vi "Solve2.vi"(8 "Error In":errorcluster, 11 "object in":refnum<class "2024_11.lvclass">) -> (0 "Error Out":errorcluster, 2 "Result":u64, 3 "object out":refnum<class "2024_11.lvclass">)   [LabVIEW 2023, in "2024_11.lvclass"]
uses:
  2024_11.lvclass
  2024_11.lvclass/2024_11.ctl
panel:
  out "x-y":u32
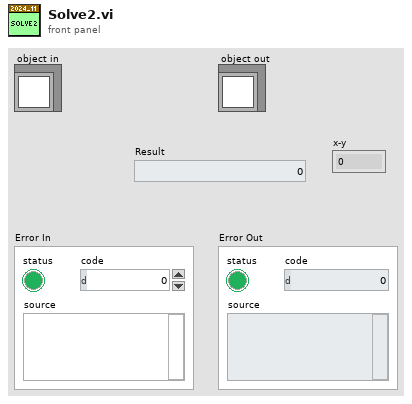
[diagram p1: front panel]
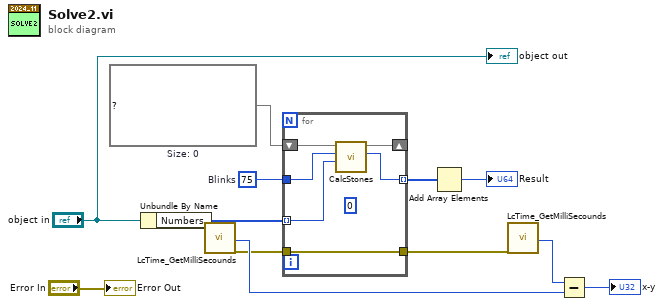
[diagram p0: block diagram]
diagram:
  w6 = 75  # Blinks
  w7 = map{cluster{"Number":u64, "Blinks":i32}, u64} {}  # Size: 0
  n1 = Unbundle By Name("object in") -> ("Numbers"=w10:u64[])
  n2 = call <userlib>:"LcTime_GetMilliSecounds.vi"() -> ("msValue"=w4:u32, "error out"=w2:errorcluster)  [unwired: 18 in]
  n3 = for {
    tunnel: w10 -> [w17] mode=indexing
    tunnel: [w15] -> w8 mode=indexing
    shift-right: [w16] -> _
    shift-left: w7 -> [w18]
    tunnel: w6 -> [w14]
    tunnel: w2 -> [w13]
    tunnel: [w13] -> w1
    (unwired) 0
    n4 = call "CalcStones.vi"("StoneNumber"=w17, "BlinkNumber(n-0)"=w14, "DataIn"=w18) -> ("NumberOfStones"=w15:u64, "DataOut"=w16:map{cluster{"Number":u64, "Blinks":i32}, u64})  [unwired: 7 in]
  }
  n5 = Add Array Elements(numeric array=w8) -> (sum=→"Result":u64)
  n6 = call <userlib>:"LcTime_GetMilliSecounds.vi"("error in (no error)"=w1) -> ("msValue"=w5:u32)  [unwired: 17 in, 1 out]
  n7 = Subtract(x=w5, y=w4) -> (x-y=→"x-y":u32)
  "Error Out" <- "Error In"
  "object out" <- "object in"
